vi "曲线对齐.vi"() -> ()   [LabVIEW 2015]
uses:
  <vilib>/Utility/miscctls.llb/LVCursorListTypeDef.ctl
  <vilib>/Utility/file.llb/Read Delimited Spreadsheet (DBL).vi
  <vilib>/gmath/NI_Gmath.lvlib
panel:
  in  "重采样间隔":dbl=0.1 format="%.3fs"
  in  "取消修改":bool
  in  "当前编辑曲线":T1
  in  "确认修改":bool
  in  "功能选择":T2
  in  "加载数据":bool
  out "曲线对齐":cluster{"理论时间":dbl[], "力":dbl[]}[](graph)
  out "all rows 2":dbl[][](array[numeric]) caption="所有行"
  in  "理论曲线路径":path=path "D:/曲线处理/理论1.csv" caption="理论"
  out "all rows":dbl[][](array[numeric]) caption="所有行"
  in  "测量曲线路径":path=path "D:/曲线处理/实测1.csv" caption="实际"
  in  "Enqueue Element":bool caption="元素入队列"
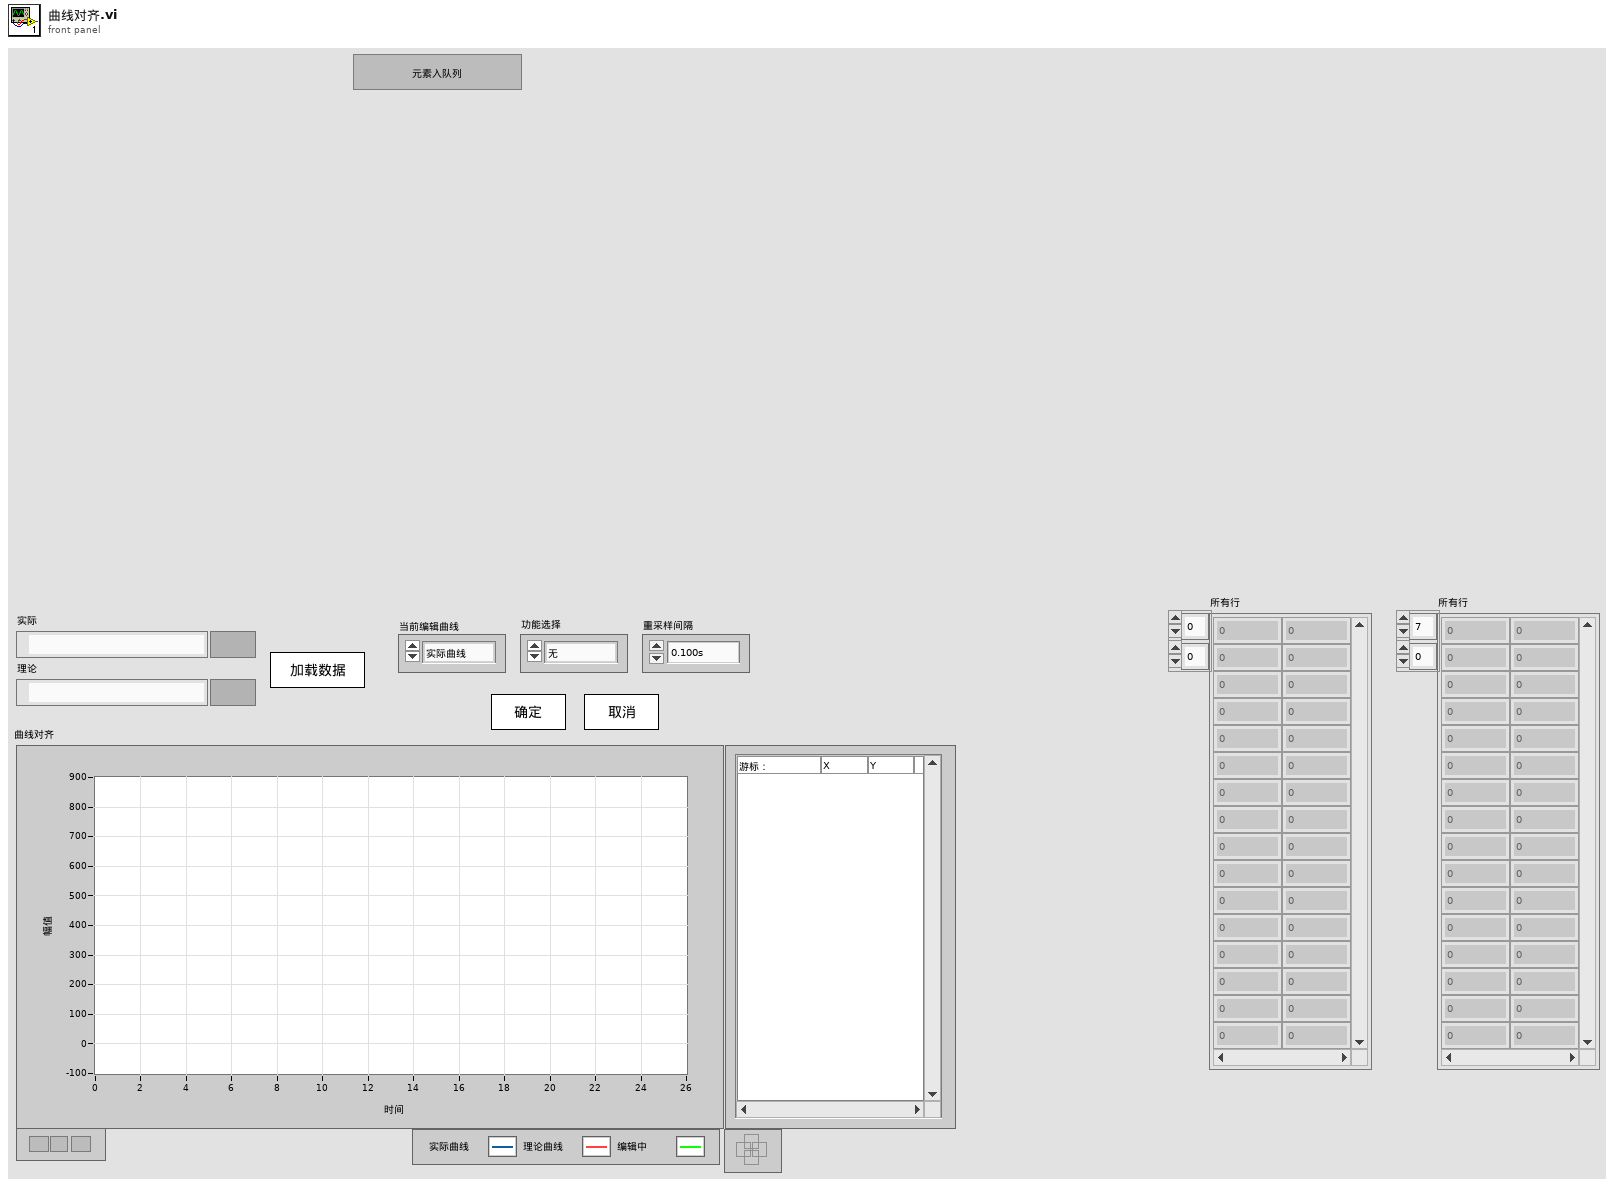
[diagram p1: front panel]
types:
  T1 = typedef "曲线选择.ctl" = enum16{"实际曲线", "理论曲线", "编辑中曲线", "实际曲线原始值", "理论曲线原始值"}
  T2 = typedef "功能选择.ctl" = enum16{"无", "缩放曲线", "剪裁曲线", "对齐曲线", "初始值置0", "重采样", "曲线平滑"}
  T3 = typedef "LVCursorListTypeDef.ctl" = cluster{"Name":string, "Color":u32, "Style":u8, "Point Style":u8, "Name Visible":bool, "Allow Drag":bool, "Cursor Mode":u32, "Plot":i32, "Index":i32, "Position":cluster{"X":dbl, "Y":dbl}, "X Scale":u32, "Y Scale":u32, "Watch Plots":i32[], "Watch All Plots":bool, "Plot Area":i32, "Label Offset":cluster{"X":dbl, "Y":dbl}}[]
  T4 = cluster{"Name":string, "Color":u32, "Style":u8, "Point Style":u8, "Name Visible":bool, "Allow Drag":bool, "Cursor Mode":u32, "Plot":i32, "Index":i32, "Position":cluster{"X":dbl, "Y":dbl}, "X Scale":u32, "Y Scale":u32, "Watch Plots":i32[], "Watch All Plots":bool, "Plot Area":i32, "Label Offset":cluster{"X":dbl, "Y":dbl}}
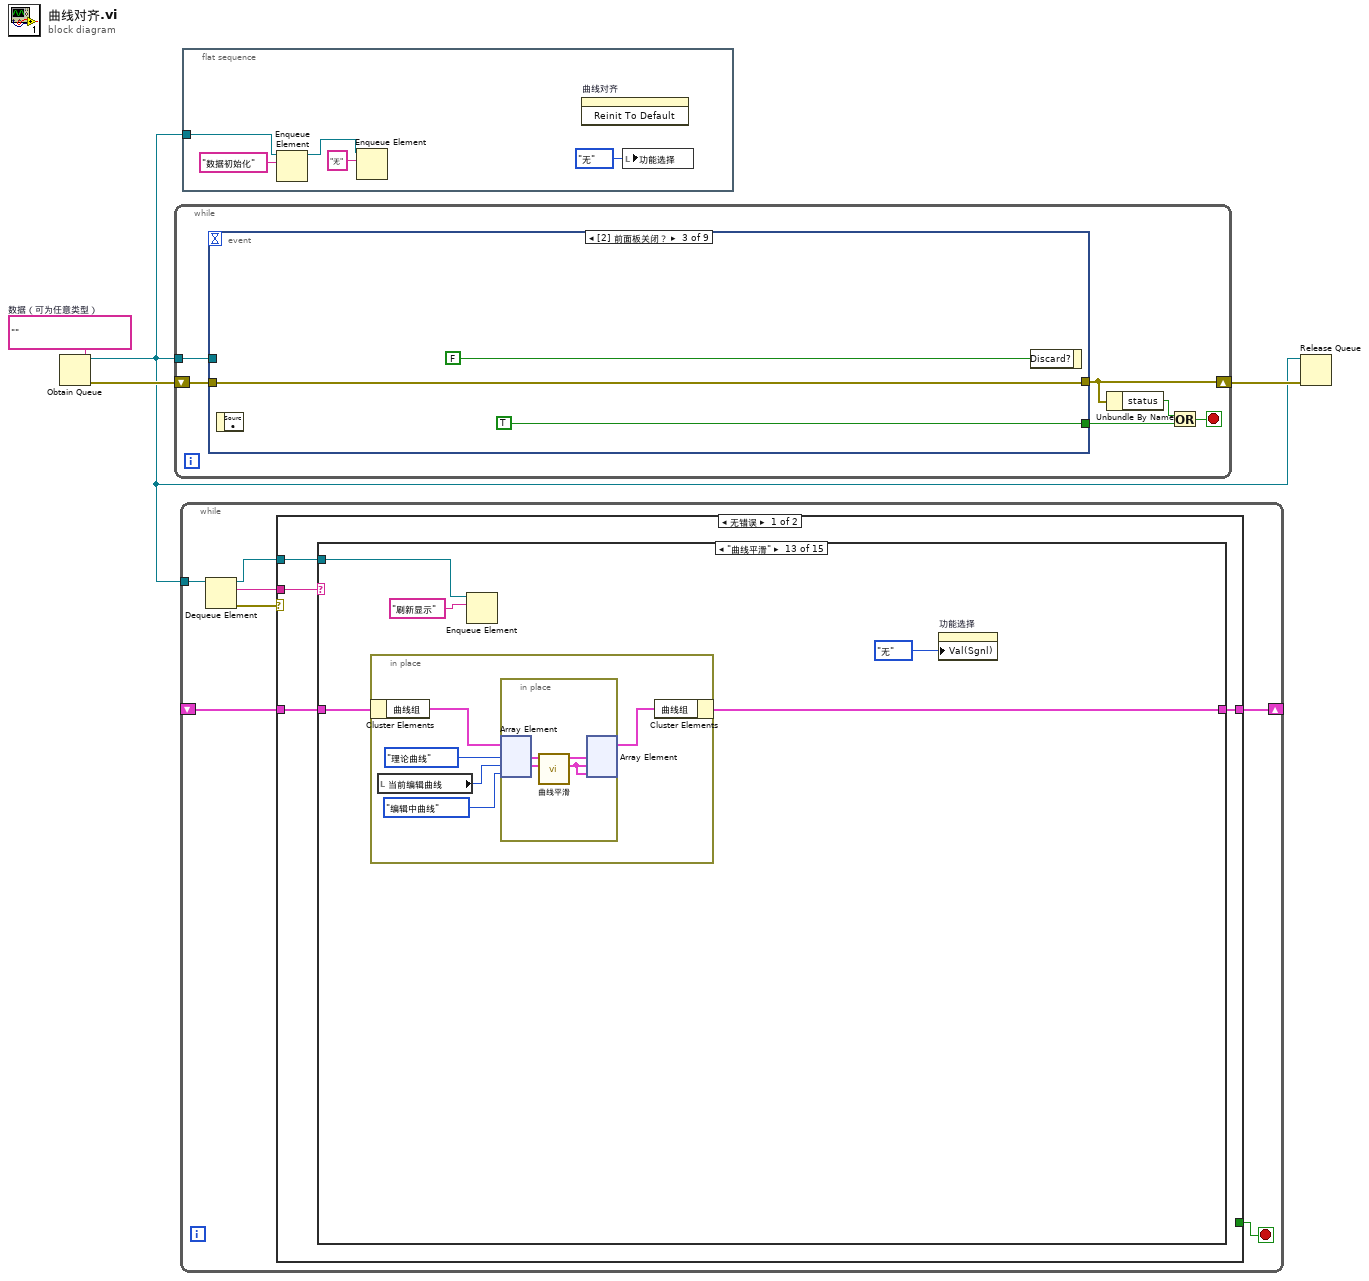
[diagram p0: block diagram]
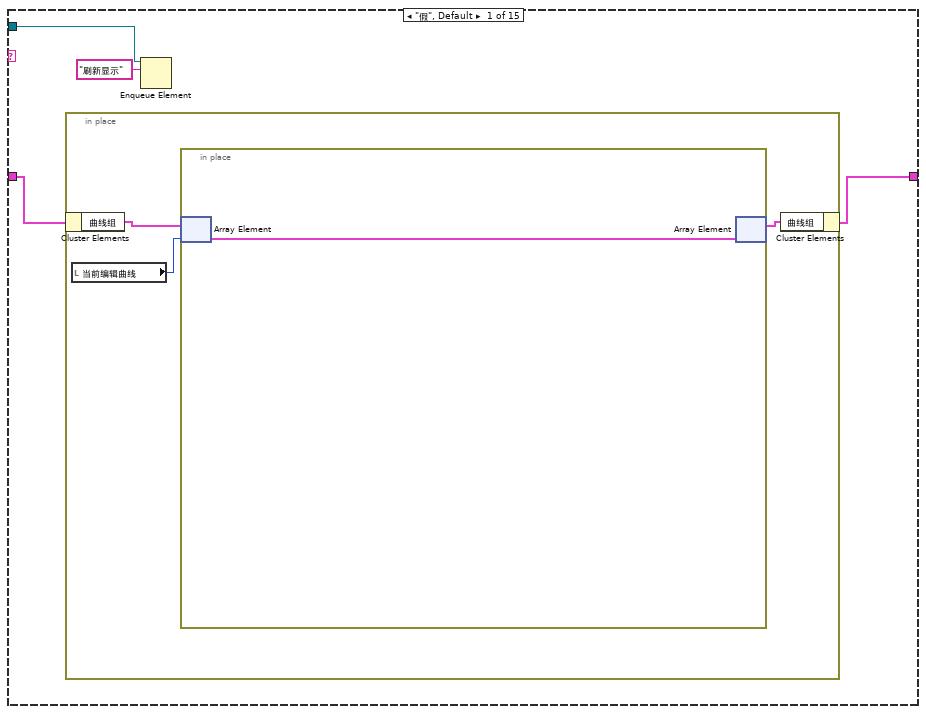
[diagram p2: hidden frame]
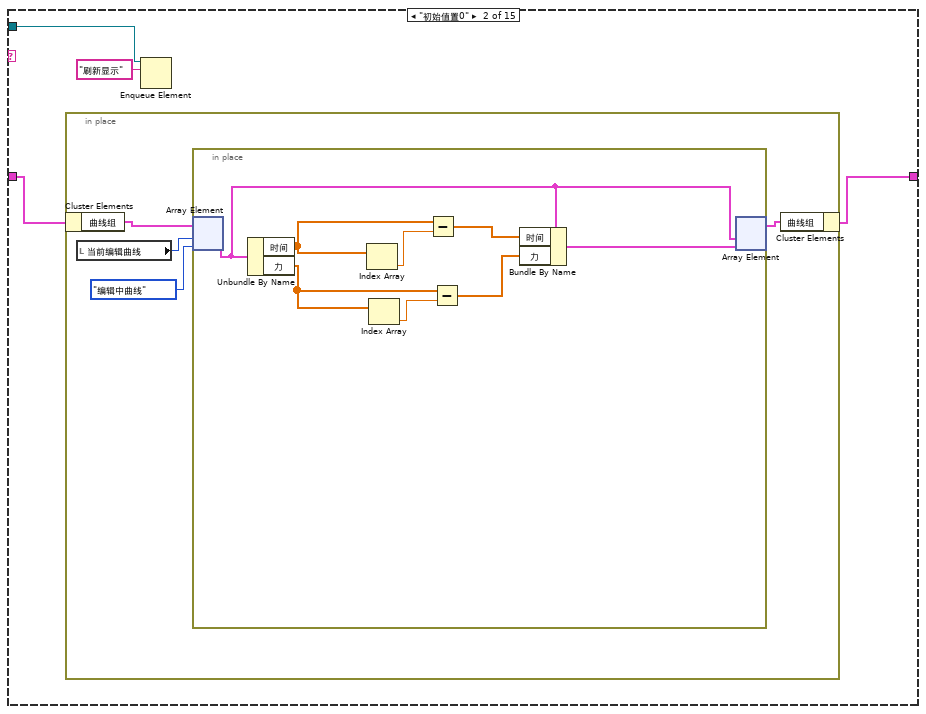
[diagram p3: hidden frame]
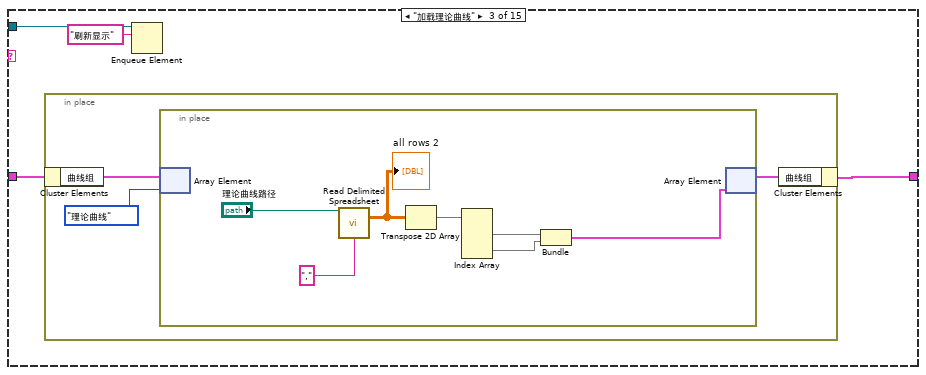
[diagram p4: hidden frame]
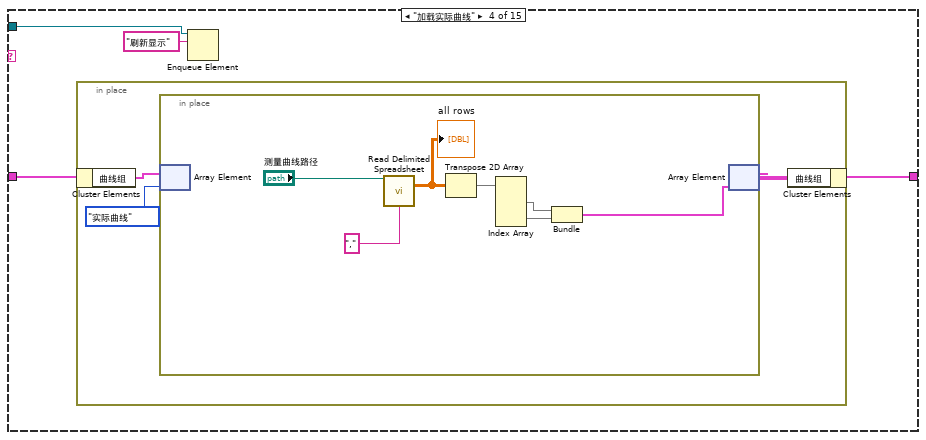
[diagram p5: hidden frame]
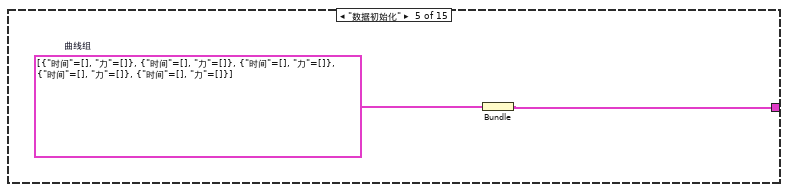
[diagram p6: hidden frame]
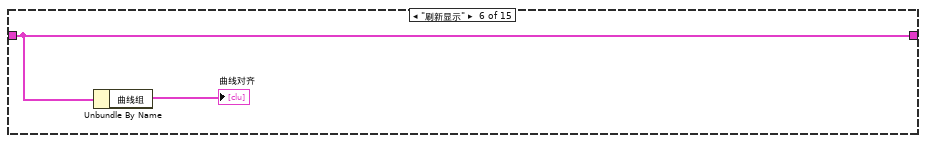
[diagram p7: hidden frame]
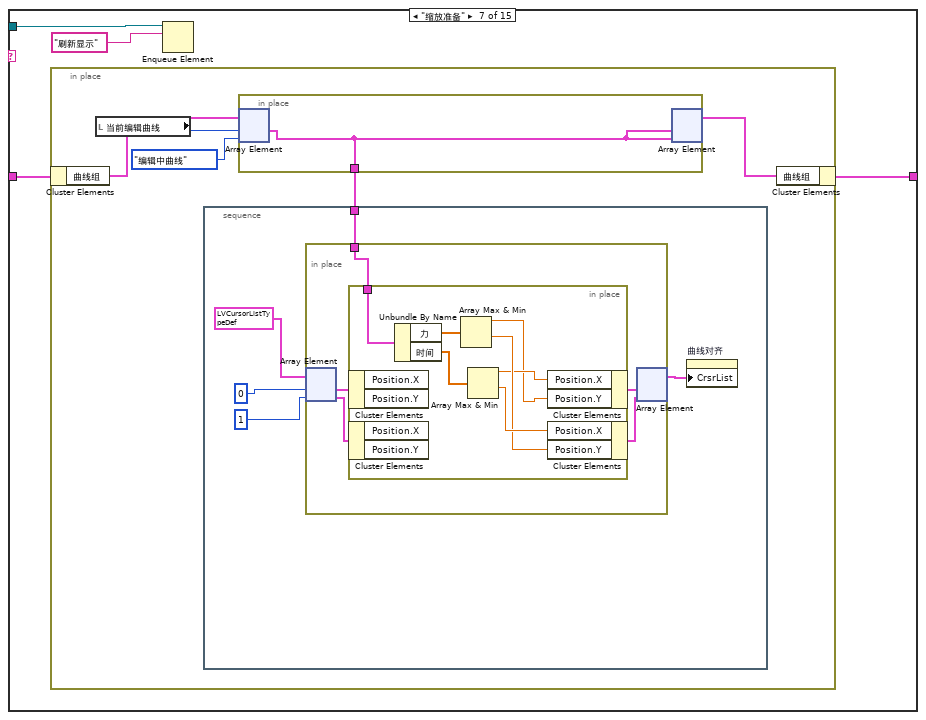
[diagram p8: hidden frame]
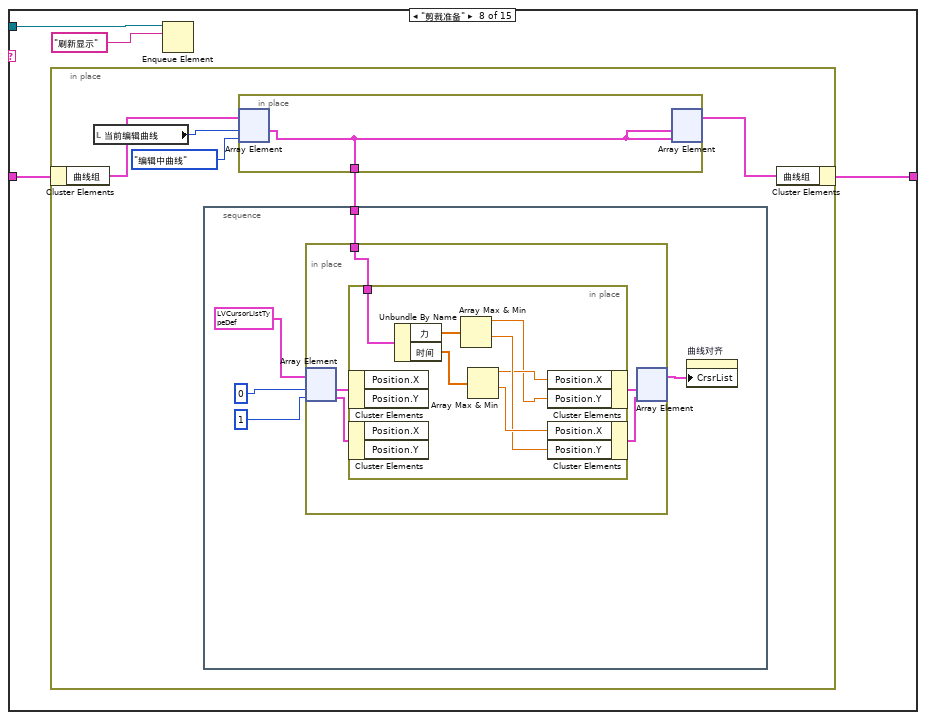
[diagram p9: hidden frame]
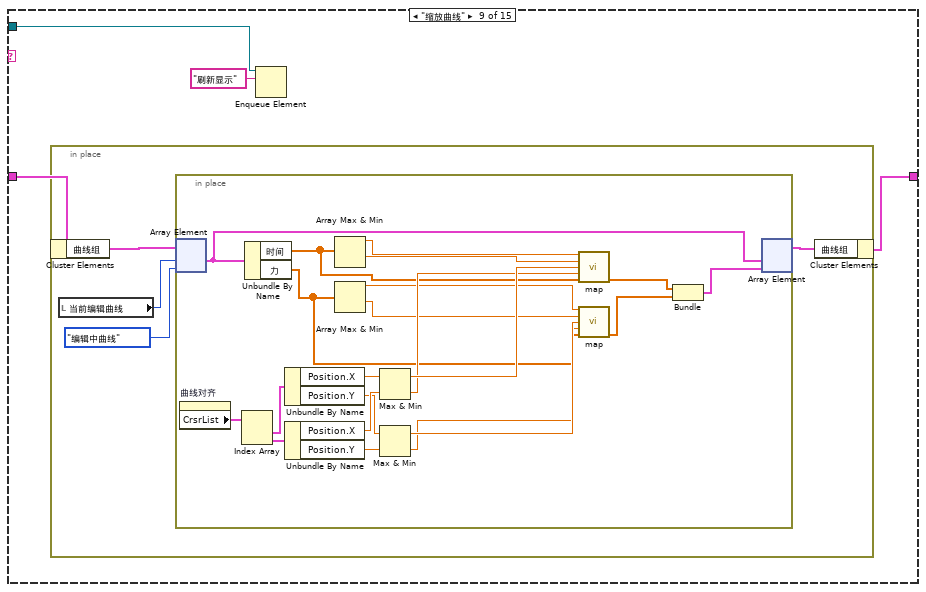
[diagram p10: hidden frame]
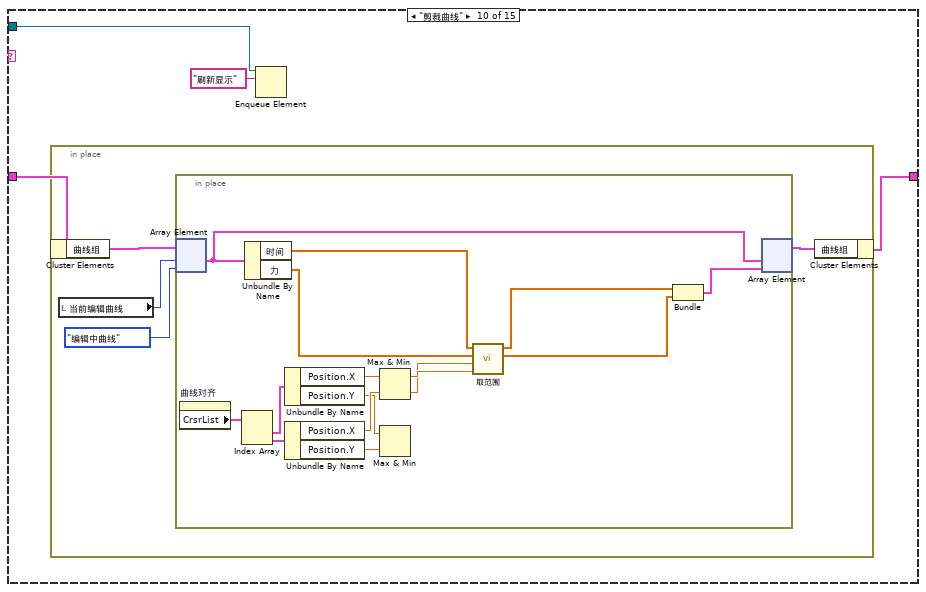
[diagram p11: hidden frame]
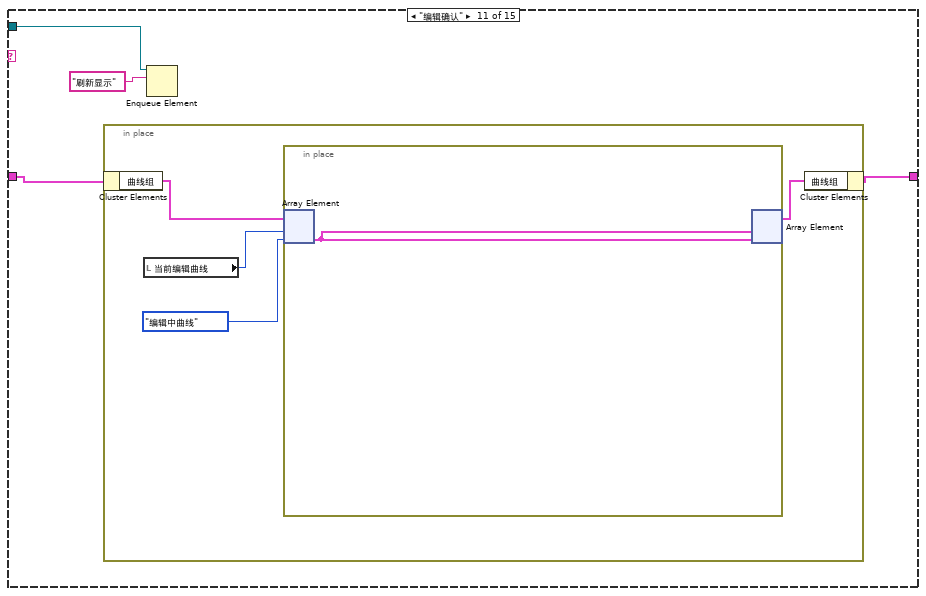
[diagram p12: hidden frame]
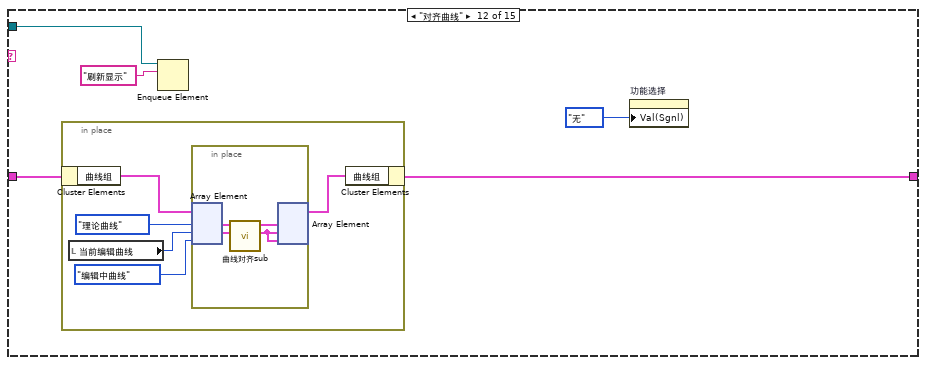
[diagram p13: hidden frame]
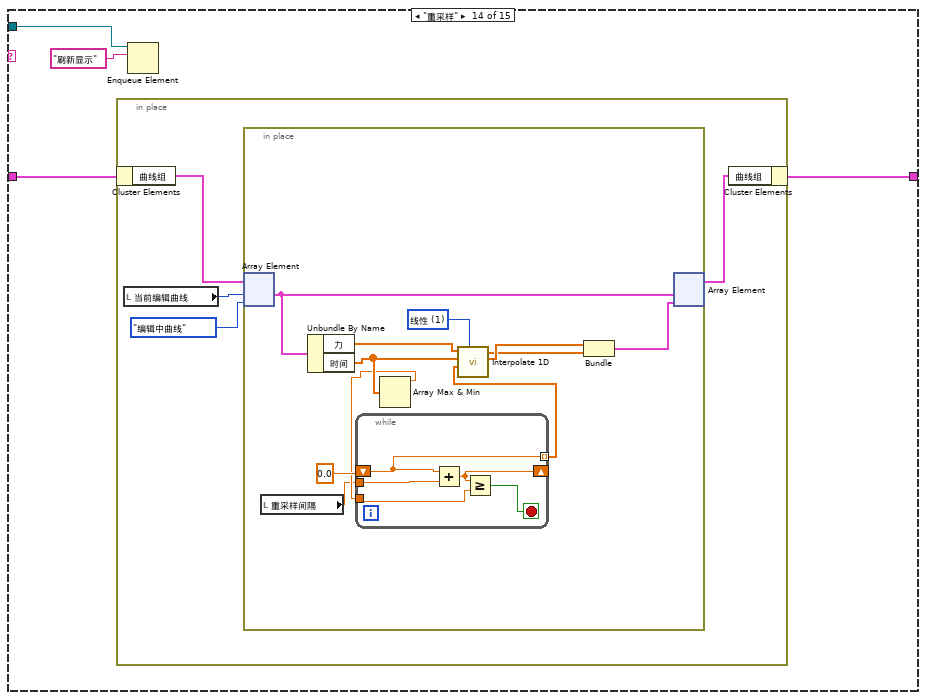
[diagram p14: hidden frame]
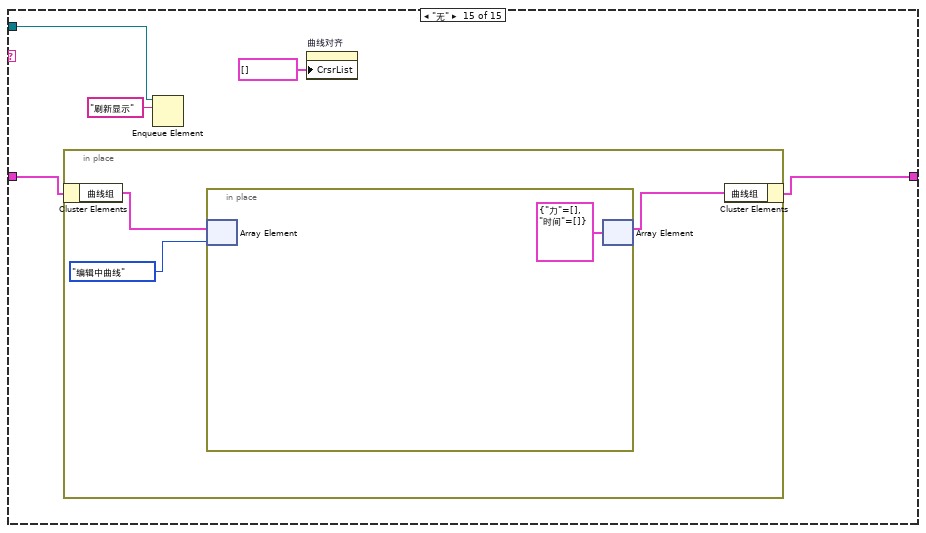
[diagram p15: hidden frame]
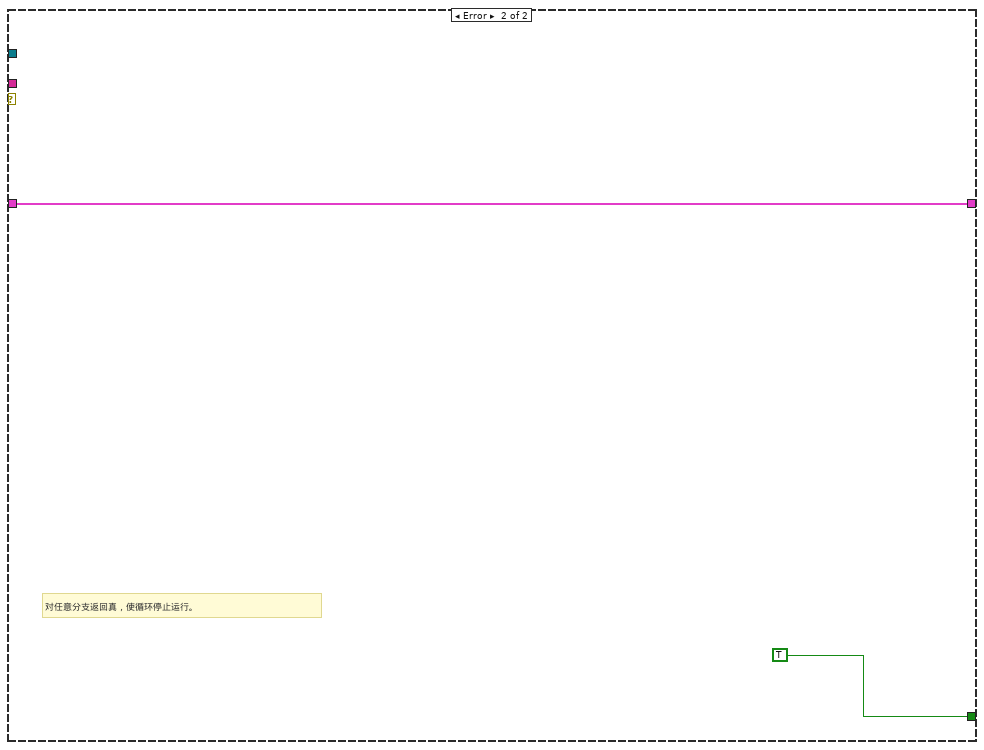
[diagram p16: hidden frame]
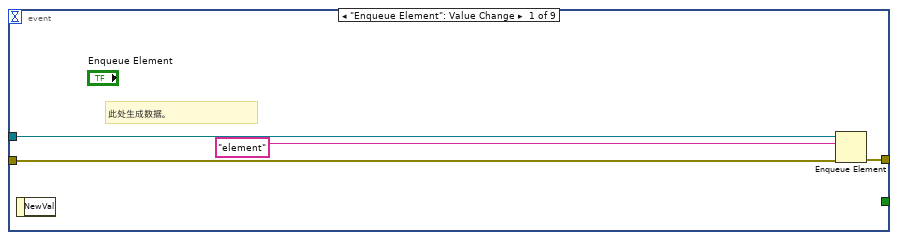
[diagram p17: hidden frame]
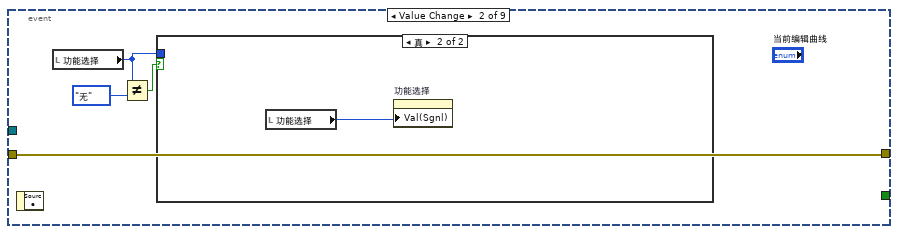
[diagram p18: hidden frame]
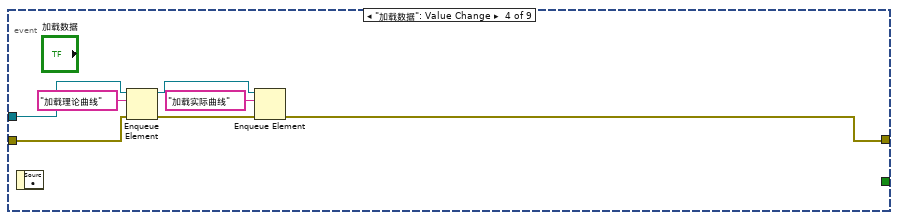
[diagram p20: hidden frame]
diagram:
  w4 = ""  # 数据（可为任意类型）
  n1 = Obtain Queue(element data type=w4) -> (queue out=w1:refnum<queue>, error out=w2:errorcluster)  [unwired: 4 in, 1 out]
  n2 = while {
    shift-right: [w6] -> w3
    shift-left: w2 -> [w9]
    tunnel: w1 -> [w10]
    stop <- w7 stop-if-true
    n3 = event shown="[2] 前面板关闭？" {
      selector: _ -> [_ _ _ _ _ _ _ _ _]
      dyn-events: _ -> [_ _ _ _ _ _ _ _ _]
      timeout: _ -> [_ _ _ _ _ _ _ _ _]
      tunnel: w10 -> [w14 _ _ w27 w33 _ w43 w47 w64]
      tunnel: w9 -> [w13 w18 w22 w24 w34 w38 w44 w49 w66]
      tunnel: [w12 w18 w22 w23 w34 w37 w44 w49 w66] -> w6
      tunnel: [_ _ TRUE ("stop") _ _ _ _ _ _] -> w8
      event "Enqueue Element": Value Change {
        # "此处生成数据。"
        n4 = event-data() -> ()  [unwired: 1 in, 1 out]
        n5 = Enqueue Element(queue=w14, element="element", error in (no error)=w13) -> (error out=w12:errorcluster)  [unwired: 1 in, 2 out]
      }
      event Value Change {
        n6 = event-data() -> ()  [unwired: 1 in, 1 out]
        n7 = local read "功能选择"() -> (w15:T2)
        n8 = Not Equal?(x=w15, y=功能选择."无") -> (x != y?=w17:bool)
        n9 = case shown="真" w17 {
          tunnel: w15 -> [_ _]
          frame False {
          }
          frame True {
            n10 = local read "功能选择"() -> (w19:T2)
            n11 = property on="功能选择" class="Enum (严格)"("Val(Sgnl)"=w19) -> ()  [unwired: 2 in, 2 out]
          }
        }
      }
      event Panel Close? {
        n12 = event-data() -> ()  [unwired: 1 in, 1 out]
        n13 = event-data("Discard?"=FALSE ("放弃？")) -> ()  [unwired: 1 in, 1 out]
      }
      event "加载数据": Value Change {
        n14 = event-data() -> ()  [unwired: 1 in, 1 out]
        n15 = Enqueue Element(queue=w27, element="加载理论曲线" ("元素"), error in (no error)=w24) -> (queue out=w26:refnum<queue>, error out=w25:errorcluster)  [unwired: 1 in, 1 out]
        n16 = Enqueue Element(queue=w26, element="加载实际曲线" ("元素"), error in (no error)=w25) -> (error out=w23:errorcluster)  [unwired: 1 in, 2 out]
      }
      event "确认修改": Value Change {
        n17 = event-data() -> ()  [unwired: 1 in, 1 out]
        n18 = local read "功能选择"() -> (w32:T2)
        n19 = Not Equal?(x=w32, y=功能选择."无") -> (x != y?=w31:bool)
        n20 = case shown="真" w31 {
          tunnel: w33 -> [_ w35]
          frame False {
          }
          frame True {
            n21 = Enqueue Element(queue=w35, element="编辑确认" ("元素")) -> ()  [unwired: 2 in, 3 out]
          }
        }
      }
      event "取消修改": Value Change {
        n22 = event-data() -> ()  [unwired: 1 in, 1 out]
        n23 = property on="功能选择" class="Enum (严格)"(error in=w38, "Val(Sgnl)"=功能选择."无" ("值(信号)")) -> (error out=w37:errorcluster)  [unwired: 1 in, 1 out]
      }
      event "重采样间隔": Value Change {
        n24 = event-data() -> ()  [unwired: 1 in, 1 out]
        n25 = local read "功能选择"() -> (w41:T2)
        n26 = Equal?(x=w41, y=功能选择."重采样") -> (x = y?=w42:bool)
        n27 = case shown="真" w42 {
          tunnel: w43 -> [_ w45]
          frame False {
          }
          frame True {
            n28 = Enqueue Element(queue=w45, element="重采样" ("元素")) -> ()  [unwired: 2 in, 3 out]
          }
        }
      }
      event Value Change {
        n29 = event-data() -> ("NewVal"=w48:T2)  [unwired: 1 in]
        n30 = case shown="\"曲线平滑\"" w48 {
          tunnel: w47 -> [w50 w53 w54 w56 w58 w61 w62]
          frame "缩放曲线", Default {
            n31 = Enqueue Element(queue=w50, element="缩放准备" ("元素")) -> ()  [unwired: 2 in, 3 out]
          }
          frame "无" {
            n32 = Enqueue Element(queue=w53, element="无" ("元素")) -> ()  [unwired: 2 in, 3 out]
          }
          frame "剪裁曲线" {
            n33 = Enqueue Element(queue=w54, element="剪裁准备" ("元素")) -> ()  [unwired: 2 in, 3 out]
          }
          frame "对齐曲线" {
            n34 = Enqueue Element(queue=w56, element="对齐曲线" ("元素")) -> ()  [unwired: 2 in, 3 out]
          }
          frame "初始值置0" {
            n35 = Enqueue Element(queue=w58, element="初始值置0" ("元素")) -> ()  [unwired: 2 in, 3 out]
          }
          frame "重采样" {
            n36 = Enqueue Element(queue=w61, element="重采样" ("元素")) -> ()  [unwired: 2 in, 3 out]
          }
          frame "曲线平滑" {
            n37 = Enqueue Element(queue=w62, element="曲线平滑" ("元素")) -> ()  [unwired: 2 in, 3 out]
          }
        }
      }
      event "曲线对齐": Cursor Move {
        n38 = event-data() -> ()  [unwired: 1 in, 8 out]
        n39 = local read "功能选择"() -> (w65:T2)
        n40 = case shown="\"无\", 默认" w65 {
          tunnel: w64 -> [_ w67 w69]
          frame "无", Default {
          }
          frame "缩放曲线" {
            n41 = Enqueue Element(queue=w67, element="缩放曲线" ("元素")) -> ()  [unwired: 2 in, 3 out]
          }
          frame "剪裁曲线" {
            n42 = Enqueue Element(queue=w69, element="剪裁曲线" ("元素")) -> ()  [unwired: 2 in, 3 out]
          }
        }
      }
    }
    n43 = Unbundle By Name(w6) -> ("status"=w5:bool)
    n44 = Or(x=w5, y=w8) -> (x .or. y?=w7:bool)
  }
  n45 = while {
    tunnel: w1 -> [w72]
    shift-right: [w74] -> _
    shift-left: _ -> [w73]
    stop <- w75 stop-if-true
    n46 = Dequeue Element(queue=w72) -> (queue out=w71:refnum<queue>, element=w76:string, error out=w77:errorcluster)  [unwired: 2 in, 1 out]
    n47 = case shown="无错误" w77 {
      tunnel: w76 -> [w81 _]
      tunnel: [_ TRUE] -> w75
      tunnel: [w78 w314] -> w74
      tunnel: w73 -> [w80 w314]
      tunnel: w71 -> [w79 _]
      frame No Error {
        n48 = case shown="\"曲线平滑\"" w81 {
          tunnel: [w82 w90 w109 w123 w135 w137 w138 w165 w192 w221 w244 w256 w270 w283 w305] -> w78
          tunnel: w80 -> [w83 w91 w106 w120 _ w137 w139 w166 w193 w222 w245 w257 w271 w284 w306]
          tunnel: w79 -> [w84 w92 w108 w121 _ _ w140 w167 w194 w223 w246 w254 w268 w281 w307]
          frame "假", Default {
            n49 = in-place {
              n50 = in-place-cluster #1(w83) -> ("曲线组"=w88:cluster{"时间":dbl[], "力":dbl[]}[])
              n51 = local read "当前编辑曲线"() -> (w86:T1)
              n52 = in-place {
                n53 = in-place-array #2(w88, w86) -> (w89:cluster{"时间":dbl[], "力":dbl[]})
                n54 = in-place-array #2(w89) -> (w87:cluster{"时间":dbl[], "力":dbl[]}[])  [unwired: 1 out]
              }
              n55 = in-place-cluster #1("曲线组"=w87) -> (w82:cluster{"曲线组":cluster{"时间":dbl[], "力":dbl[]}[]})
            }
            n56 = Enqueue Element(queue=w84, element="刷新显示" ("元素")) -> ()  [unwired: 2 in, 3 out]
          }
          frame "初始值置0" {
            n57 = in-place {
              n58 = in-place-cluster #3(w91) -> ("曲线组"=w97:cluster{"时间":dbl[], "力":dbl[]}[])
              n59 = local read "当前编辑曲线"() -> (w95:T1)
              n60 = in-place {
                n61 = in-place-array #4(w97, w95, 曲线选择."编辑中曲线" ("当前编辑曲线")) -> (w99:cluster{"时间":dbl[], "力":dbl[]})  [unwired: 1 out]
                n62 = Unbundle By Name(w99) -> ("时间"=w105:dbl[], "力"=w103:dbl[])
                n63 = Index Array(array=w105) -> (element=w104:dbl)  [unwired: 1 in]
                n64 = Index Array(array=w103) -> (element=w102:dbl)  [unwired: 1 in]
                n65 = Subtract(x=w105, y=w104) -> (x-y=w101:dbl[])
                n66 = Subtract(x=w103, y=w102) -> (x-y=w100:dbl[])
                n67 = Bundle By Name(cluster=w99, "时间"=w101, "力"=w100) -> (w98:cluster{"时间":dbl[], "力":dbl[]})
                n68 = in-place-array #4(w99, w98) -> (w96:cluster{"时间":dbl[], "力":dbl[]}[])  [unwired: 2 out]
              }
              n69 = in-place-cluster #3("曲线组"=w96) -> (w90:cluster{"曲线组":cluster{"时间":dbl[], "力":dbl[]}[]})
            }
            n70 = Enqueue Element(queue=w92, element="刷新显示" ("元素")) -> ()  [unwired: 2 in, 3 out]
          }
          frame "加载理论曲线" {
            n71 = in-place {
              n72 = in-place-cluster #5(w106) -> ("曲线组"=w112:cluster{"时间":dbl[], "力":dbl[]}[])
              n73 = in-place {
                n74 = in-place-array #6(w112, 曲线选择."理论曲线" ("当前编辑曲线")) -> ()  [unwired: 1 out]
                n75 = call-poly <vilib>:"Read Delimited Spreadsheet.vi"("file path (dialog if empty)"="理论曲线路径", "delimiter (\\t)"="," ("delimiter (\\t)")) -> ("all rows"=w116:dbl[][])  [unwired: 8 in, 5 out]
                "all rows 2" <- w116
                n76 = Transpose 2D Array(2D array=w116) -> (transposed array=w117:dbl[][])
                n77 = Index Array(array=w117) -> (element #1=w115:dbl[], element #2=w114:dbl[])  [unwired: 4 in]
                n78 = Bundle(w115, w114) -> (w113:cluster{dbl[], dbl[]})  [unwired: 1 in]
                n79 = in-place-array #6(w113) -> (w111:cluster{"时间":dbl[], "力":dbl[]}[])  [unwired: 1 out]
              }
              n80 = in-place-cluster #5("曲线组"=w111) -> (w109:cluster{"曲线组":cluster{"时间":dbl[], "力":dbl[]}[]})
            }
            n81 = Enqueue Element(queue=w108, element="刷新显示" ("元素")) -> ()  [unwired: 2 in, 3 out]
          }
          frame "加载实际曲线" {
            n82 = in-place {
              n83 = in-place-cluster #7(w120) -> ("曲线组"=w126:cluster{"时间":dbl[], "力":dbl[]}[])
              n84 = in-place {
                n85 = in-place-array #8(w126, 曲线选择."实际曲线") -> ()  [unwired: 1 out]
                n86 = call-poly <vilib>:"Read Delimited Spreadsheet.vi"("file path (dialog if empty)"="测量曲线路径", "delimiter (\\t)"="," ("delimiter (\\t)")) -> ("all rows"=w132:dbl[][])  [unwired: 8 in, 5 out]
                "all rows" <- w132
                n87 = Transpose 2D Array(2D array=w132) -> (transposed array=w133:dbl[][])
                n88 = Index Array(array=w133) -> (element #1=w129:dbl[], element #2=w128:dbl[])  [unwired: 4 in]
                n89 = Bundle(w129, w128) -> (w127:cluster{dbl[], dbl[]})  [unwired: 1 in]
                n90 = in-place-array #8(w127) -> (w124:cluster{"时间":dbl[], "力":dbl[]}[])  [unwired: 1 out]
              }
              n91 = in-place-cluster #7("曲线组"=w124) -> (w123:cluster{"曲线组":cluster{"时间":dbl[], "力":dbl[]}[]})
            }
            n92 = Enqueue Element(queue=w121, element="刷新显示" ("元素")) -> ()  [unwired: 2 in, 3 out]
          }
          frame "数据初始化" {
            w134 = cluster{"时间":dbl[], "力":dbl[]}[] [{"时间"=[], "力"=[]}, {"时间"=[], "力"=[]}, {"时间"=[], "力"=[]}, {"时间"=[], "力"=[]}, {"时间"=[], "力"=[]}]  # 曲线组
            n93 = Bundle("曲线组"=w134) -> (w135:cluster{"曲线组":cluster{"时间":dbl[], "力":dbl[]}[]})  [unwired: 1 in]
          }
          frame "刷新显示" {
            n94 = Unbundle By Name(w137) -> ("曲线组"=→"曲线对齐":cluster{"时间":dbl[], "力":dbl[]}[])
          }
          frame "缩放准备" {
            n95 = in-place {
              n96 = in-place-cluster #9(w139) -> ("曲线组"=w146:cluster{"时间":dbl[], "力":dbl[]}[])
              n97 = local read "当前编辑曲线"() -> (w142:T1)
              n98 = in-place {
                in-place-border: [w147] -> w143
                n99 = in-place-array #10(w146, w142, 曲线选择."编辑中曲线" ("当前编辑曲线")) -> (w147:cluster{"时间":dbl[], "力":dbl[]})  [unwired: 1 out]
                n100 = in-place-array #10(w147, w147) -> (w144:cluster{"时间":dbl[], "力":dbl[]}[])  [unwired: 2 out]
              }
              n101 = stacked-sequence {
                tunnel: w143 -> [w148]
                frame #0 {
                  n102 = in-place {
                    in-place-border: w148 -> [w153]
                    n103 = in-place-array #11(T3 [{"Name"="游标0", "Color"=16711680, "Style"=8, "Point Style"=13, "Name Visible"=FALSE, "Allow Drag"=TRUE, "Cursor Mode"=0, "Plot"=0, "Index"=0, "Position"={"X"=24.900169204737733, "Y"=876.3513513513514}, "X Scale"=0, "Y Scale"=0, "Watch Plots"=[], "Watch All Plots"=FALSE, "Plot Area"=0, "Label Offset"={"X"=0.0, "Y"=67.56756756756761}}, {"Name"="游标1", "Color"=16860, "Style"=8, "Point Style"=13, "Name Visible"=FALSE, "Allow Drag"=TRUE, "Cursor Mode"=0, "Plot"=0, "Index"=0, "Position"={"X"=-2.199661590524536, "Y"=1.3513513513513553}, "X Scale"=0, "Y Scale"=0, "Watch Plots"=[], "Watch All Plots"=FALSE, "Plot Area"=0, "Label Offset"={"X"=8.881784197001252e-16, "Y"=67.56756756756756}}] ("游标列表"), 0, 1) -> (w157:T4, w156:T4)
                    n104 = in-place {
                      in-place-border: w153 -> [w160]
                      n105 = in-place-cluster #12(w157) -> ()  [unwired: 2 out]
                      n106 = in-place-cluster #13(w156) -> ()  [unwired: 2 out]
                      n107 = Unbundle By Name(w160) -> ("力"=w159:dbl[], "时间"=w158:dbl[])
                      n108 = Array Max & Min(array=w159) -> (max value=w161:dbl, min value=w163:dbl)  [unwired: 2 out]
                      n109 = Array Max & Min(array=w158) -> (max value=w162:dbl, min value=w164:dbl)  [unwired: 2 out]
                      n110 = in-place-cluster #12("Position.X"=w162, "Position.Y"=w161) -> (w155:T4)
                      n111 = in-place-cluster #13("Position.X"=w164, "Position.Y"=w163) -> (w154:T4)
                    }
                    n112 = in-place-array #11(w155, w154) -> (w149:T3)  [unwired: 2 out]
                  }
                  n113 = property on="曲线对齐" class="XYGraph (严格)"("CrsrList"=w149) -> ()  [unwired: 2 in, 2 out]
                }
              }
              n114 = in-place-cluster #9("曲线组"=w144) -> (w138:cluster{"曲线组":cluster{"时间":dbl[], "力":dbl[]}[]})
            }
            n115 = Enqueue Element(queue=w140, element="刷新显示" ("元素")) -> ()  [unwired: 2 in, 3 out]
          }
          frame "剪裁准备" {
            n116 = in-place {
              n117 = in-place-cluster #14(w166) -> ("曲线组"=w173:cluster{"时间":dbl[], "力":dbl[]}[])
              n118 = local read "当前编辑曲线"() -> (w169:T1)
              n119 = in-place {
                in-place-border: [w174] -> w170
                n120 = in-place-array #15(w173, w169, 曲线选择."编辑中曲线" ("当前编辑曲线")) -> (w174:cluster{"时间":dbl[], "力":dbl[]})  [unwired: 1 out]
                n121 = in-place-array #15(w174, w174) -> (w171:cluster{"时间":dbl[], "力":dbl[]}[])  [unwired: 2 out]
              }
              n122 = stacked-sequence {
                tunnel: w170 -> [w175]
                frame #0 {
                  n123 = in-place {
                    in-place-border: w175 -> [w180]
                    n124 = in-place-array #16(T3 [{"Name"="游标0", "Color"=16711680, "Style"=8, "Point Style"=13, "Name Visible"=FALSE, "Allow Drag"=TRUE, "Cursor Mode"=0, "Plot"=0, "Index"=0, "Position"={"X"=24.900169204737733, "Y"=876.3513513513514}, "X Scale"=0, "Y Scale"=0, "Watch Plots"=[], "Watch All Plots"=FALSE, "Plot Area"=0, "Label Offset"={"X"=0.0, "Y"=67.56756756756761}}, {"Name"="游标1", "Color"=16860, "Style"=8, "Point Style"=13, "Name Visible"=FALSE, "Allow Drag"=TRUE, "Cursor Mode"=0, "Plot"=0, "Index"=0, "Position"={"X"=-2.199661590524536, "Y"=1.3513513513513553}, "X Scale"=0, "Y Scale"=0, "Watch Plots"=[], "Watch All Plots"=FALSE, "Plot Area"=0, "Label Offset"={"X"=8.881784197001252e-16, "Y"=67.56756756756756}}] ("游标列表"), 0, 1) -> (w184:T4, w183:T4)
                    n125 = in-place {
                      in-place-border: w180 -> [w187]
                      n126 = in-place-cluster #17(w184) -> ()  [unwired: 2 out]
                      n127 = in-place-cluster #18(w183) -> ()  [unwired: 2 out]
                      n128 = Unbundle By Name(w187) -> ("力"=w186:dbl[], "时间"=w185:dbl[])
                      n129 = Array Max & Min(array=w186) -> (max value=w188:dbl, min value=w190:dbl)  [unwired: 2 out]
                      n130 = Array Max & Min(array=w185) -> (max value=w189:dbl, min value=w191:dbl)  [unwired: 2 out]
                      n131 = in-place-cluster #17("Position.X"=w189, "Position.Y"=w188) -> (w182:T4)
                      n132 = in-place-cluster #18("Position.X"=w191, "Position.Y"=w190) -> (w181:T4)
                    }
                    n133 = in-place-array #16(w182, w181) -> (w176:T3)  [unwired: 2 out]
                  }
                  n134 = property on="曲线对齐" class="XYGraph (严格)"("CrsrList"=w176) -> ()  [unwired: 2 in, 2 out]
                }
              }
              n135 = in-place-cluster #14("曲线组"=w171) -> (w165:cluster{"曲线组":cluster{"时间":dbl[], "力":dbl[]}[]})
            }
            n136 = Enqueue Element(queue=w167, element="刷新显示" ("元素")) -> ()  [unwired: 2 in, 3 out]
          }
          frame "缩放曲线" {
            n137 = in-place {
              n138 = in-place-cluster #19(w193) -> ("曲线组"=w199:cluster{"时间":dbl[], "力":dbl[]}[])
              n139 = local read "当前编辑曲线"() -> (w198:T1)
              n140 = in-place {
                n141 = in-place-array #20(w199, w198, 曲线选择."编辑中曲线" ("当前编辑曲线")) -> (w202:cluster{"时间":dbl[], "力":dbl[]})  [unwired: 1 out]
                n142 = property on="曲线对齐" class="XYGraph (严格)"() -> ("CrsrList"=w220:T3)  [unwired: 2 in, 2 out]
                n143 = Index Array(array=w220) -> (element #1=w219:T4, element #2=w218:T4)  [unwired: 2 in]
                n144 = Unbundle By Name(w202) -> ("时间"=w201:dbl[], "力"=w200:dbl[])
                n145 = Unbundle By Name(w219) -> ("Position.X"=w217:dbl, "Position.Y"=w215:dbl)
                n146 = Unbundle By Name(w218) -> ("Position.X"=w216:dbl, "Position.Y"=w214:dbl)
                n147 = Array Max & Min(array=w201) -> (max value=w213:dbl, min value=w212:dbl)  [unwired: 2 out]
                n148 = Array Max & Min(array=w200) -> (max value=w209:dbl, min value=w208:dbl)  [unwired: 2 out]
                n149 = Max & Min(x=w217, y=w216) -> (max(x,y)=w211:dbl, min(x,y)=w210:dbl)
                n150 = Max & Min(x=w215, y=w214) -> (max(x,y)=w207:dbl, min(x,y)=w206:dbl)
                n151 = call "map.vi"("inmax"=w213, "inmin"=w212, "outmax"=w211, "outmin"=w210, "in"=w201) -> ("out"=w205:dbl[])  [unwired: 10 in]
                n152 = call "map.vi"("inmax"=w209, "inmin"=w208, "outmax"=w207, "outmin"=w206, "in"=w200) -> ("out"=w204:dbl[])  [unwired: 10 in]
                n153 = Bundle("out"=w205, "out"=w204) -> (w203:cluster{"out":dbl[], "out":dbl[]})  [unwired: 1 in]
                n154 = in-place-array #20(w202, w203) -> (w196:cluster{"时间":dbl[], "力":dbl[]}[])  [unwired: 2 out]
              }
              n155 = in-place-cluster #19("曲线组"=w196) -> (w192:cluster{"曲线组":cluster{"时间":dbl[], "力":dbl[]}[]})
            }
            n156 = Enqueue Element(queue=w194, element="刷新显示" ("元素")) -> ()  [unwired: 2 in, 3 out]
          }
          frame "剪裁曲线" {
            n157 = in-place {
              n158 = in-place-cluster #21(w222) -> ("曲线组"=w228:cluster{"时间":dbl[], "力":dbl[]}[])
              n159 = local read "当前编辑曲线"() -> (w227:T1)
              n160 = in-place {
                n161 = in-place-array #22(w228, w227, 曲线选择."编辑中曲线" ("当前编辑曲线")) -> (w236:cluster{"时间":dbl[], "力":dbl[]})  [unwired: 1 out]
                n162 = property on="曲线对齐" class="XYGraph (严格)"() -> ("CrsrList"=w243:T3)  [unwired: 2 in, 2 out]
                n163 = Index Array(array=w243) -> (element #1=w242:T4, element #2=w241:T4)  [unwired: 2 in]
                n164 = Unbundle By Name(w236) -> ("时间"=w233:dbl[], "力"=w232:dbl[])
                n165 = Unbundle By Name(w242) -> ("Position.X"=w240:dbl, "Position.Y"=w238:dbl)
                n166 = Unbundle By Name(w241) -> ("Position.X"=w239:dbl, "Position.Y"=w237:dbl)
                n167 = Max & Min(x=w240, y=w239) -> (max(x,y)=w235:dbl, min(x,y)=w234:dbl)
                n168 = Max & Min(x=w238, y=w237) -> ()  [unwired: 2 out]
                n169 = call "取范围.vi"("max"=w235, "min"=w234, "y"=w232, "x"=w233) -> ("y"=w230:dbl[], "x"=w231:dbl[])  [unwired: 6 in]
                n170 = Bundle("x"=w231, "y"=w230) -> (w229:cluster{"x":dbl[], "y":dbl[]})  [unwired: 1 in]
                n171 = in-place-array #22(w236, w229) -> (w225:cluster{"时间":dbl[], "力":dbl[]}[])  [unwired: 2 out]
              }
              n172 = in-place-cluster #21("曲线组"=w225) -> (w221:cluster{"曲线组":cluster{"时间":dbl[], "力":dbl[]}[]})
            }
            n173 = Enqueue Element(queue=w223, element="刷新显示" ("元素")) -> ()  [unwired: 2 in, 3 out]
          }
          frame "编辑确认" {
            n174 = in-place {
              n175 = in-place-cluster #23(w245) -> ("曲线组"=w251:cluster{"时间":dbl[], "力":dbl[]}[])
              n176 = local read "当前编辑曲线"() -> (w250:T1)
              n177 = in-place {
                n178 = in-place-array #24(w251, w250, 曲线选择."编辑中曲线" ("当前编辑曲线")) -> (w252:cluster{"时间":dbl[], "力":dbl[]})  [unwired: 1 out]
                n179 = in-place-array #24(w252, w252) -> (w248:cluster{"时间":dbl[], "力":dbl[]}[])  [unwired: 2 out]
              }
              n180 = in-place-cluster #23("曲线组"=w248) -> (w244:cluster{"曲线组":cluster{"时间":dbl[], "力":dbl[]}[]})
            }
            n181 = Enqueue Element(queue=w246, element="刷新显示" ("元素")) -> ()  [unwired: 2 in, 3 out]
          }
          frame "对齐曲线" {
            n182 = in-place {
              n183 = in-place-cluster #25(w257) -> ("曲线组"=w262:cluster{"时间":dbl[], "力":dbl[]}[])
              n184 = local read "当前编辑曲线"() -> (w259:T1)
              n185 = in-place {
                n186 = in-place-array #26(w262, 曲线选择."理论曲线" ("当前编辑曲线"), w259, 曲线选择."编辑中曲线" ("当前编辑曲线")) -> (w266:cluster{"时间":dbl[], "力":dbl[]}, w265:cluster{"时间":dbl[], "力":dbl[]})  [unwired: 1 out]
                n187 = call "曲线对齐sub.vi"("测量"=w265, "理论"=w266) -> ("实测"=w263:cluster{dbl[], dbl[]}, "理论"=w264:cluster{dbl[], dbl[]})  [unwired: 8 in]
                n188 = in-place-array #26(w264, w263, w263) -> (w260:cluster{"时间":dbl[], "力":dbl[]}[])  [unwired: 3 out]
              }
              n189 = in-place-cluster #25("曲线组"=w260) -> (w256:cluster{"曲线组":cluster{"时间":dbl[], "力":dbl[]}[]})
            }
            n190 = Enqueue Element(queue=w254, element="刷新显示" ("元素")) -> ()  [unwired: 2 in, 3 out]
            n191 = property on="功能选择" class="Enum (严格)"("Val(Sgnl)"=功能选择."无" ("功能选择")) -> ()  [unwired: 2 in, 2 out]
          }
          frame "曲线平滑" {
            n192 = in-place {
              n193 = in-place-cluster #27(w271) -> ("曲线组"=w276:cluster{"时间":dbl[], "力":dbl[]}[])
              n194 = local read "当前编辑曲线"() -> (w273:T1)
              n195 = in-place {
                n196 = in-place-array #28(w276, 曲线选择."理论曲线" ("当前编辑曲线"), w273, 曲线选择."编辑中曲线" ("当前编辑曲线")) -> (w280:cluster{"时间":dbl[], "力":dbl[]}, w279:cluster{"时间":dbl[], "力":dbl[]})  [unwired: 1 out]
                n197 = call "曲线平滑.vi"("测量"=w279, "理论"=w280) -> ("实测"=w277:cluster{dbl[], dbl[]}, "理论"=w278:cluster{dbl[], dbl[]})  [unwired: 8 in]
                n198 = in-place-array #28(w278, w277, w277) -> (w274:cluster{"时间":dbl[], "力":dbl[]}[])  [unwired: 3 out]
              }
              n199 = in-place-cluster #27("曲线组"=w274) -> (w270:cluster{"曲线组":cluster{"时间":dbl[], "力":dbl[]}[]})
            }
            n200 = Enqueue Element(queue=w268, element="刷新显示" ("元素")) -> ()  [unwired: 2 in, 3 out]
            n201 = property on="功能选择" class="Enum (严格)"("Val(Sgnl)"=功能选择."无" ("功能选择")) -> ()  [unwired: 2 in, 2 out]
          }
          frame "重采样" {
            n202 = in-place {
              n203 = in-place-cluster #29(w284) -> ("曲线组"=w288:cluster{"时间":dbl[], "力":dbl[]}[])
              n204 = local read "当前编辑曲线"() -> (w287:T1)
              n205 = in-place {
                w299 = 1 items=["最近", "线性", "样条", "cubic Hermite", "拉格朗日"] ("method")
                n206 = in-place-array #30(w288, w287, 曲线选择."编辑中曲线" ("当前编辑曲线")) -> (w290:cluster{"时间":dbl[], "力":dbl[]})  [unwired: 1 out]
                n207 = local read "重采样间隔"() -> (w289:dbl)
                n208 = Unbundle By Name(w290) -> ("力"=w298:dbl[], "时间"=w296:dbl[])
                n209 = Array Max & Min(array=w296) -> (max value=w295:dbl)  [unwired: 3 out]
                n210 = while {
                  shift-right: [w304] -> _
                  shift-left: 0.0 -> [w302]
                  tunnel: w295 -> [w303]
                  tunnel: [w302] -> w294 mode=indexing
                  tunnel: w289 -> [w300]
                  stop <- w301 stop-if-true
                  n211 = Add(x=w302, y=w300) -> (x+y=w304:dbl)
                  n212 = Greater Or Equal?(x=w304, y=w303) -> (x >= y?=w301:bool)
                }
                n213 = call <vilib>:"Interpolate 1D.vi"("method"=w299, "xi"=w294, "X"=w296, "Y"=w298) -> ("xi used"=w293:dbl[], "yi"=w292:dbl[])  [unwired: 5 in, 1 out]
                n214 = Bundle("xi used"=w293, "yi"=w292) -> (w291:cluster{"xi used":dbl[], "yi":dbl[]})  [unwired: 1 in]
                n215 = in-place-array #30(w290, w291) -> (w286:cluster{"时间":dbl[], "力":dbl[]}[])  [unwired: 2 out]
              }
              n216 = in-place-cluster #29("曲线组"=w286) -> (w283:cluster{"曲线组":cluster{"时间":dbl[], "力":dbl[]}[]})
            }
            n217 = Enqueue Element(queue=w281, element="刷新显示" ("元素")) -> ()  [unwired: 2 in, 3 out]
          }
          frame "无" {
            n218 = in-place {
              n219 = in-place-cluster #31(w306) -> ("曲线组"=w312:cluster{"时间":dbl[], "力":dbl[]}[])
              n220 = in-place {
                n221 = in-place-array #32(w312, 曲线选择."编辑中曲线" ("当前编辑曲线")) -> ()  [unwired: 1 out]
                n222 = in-place-array #32(cluster{"力":dbl[], "时间":dbl[]} {"力"=[], "时间"=[]} ("元素")) -> (w310:cluster{"时间":dbl[], "力":dbl[]}[])  [unwired: 1 out]
              }
              n223 = in-place-cluster #31("曲线组"=w310) -> (w305:cluster{"曲线组":cluster{"时间":dbl[], "力":dbl[]}[]})
            }
            n224 = Enqueue Element(queue=w307, element="刷新显示" ("元素")) -> ()  [unwired: 2 in, 3 out]
            n225 = property on="曲线对齐" class="XYGraph (严格)"("CrsrList"=T3 [] ("游标列表")) -> ()  [unwired: 2 in, 2 out]
          }
        }
      }
      frame Error {
        # "对任意分支返回真，使循环停止运行。"
      }
    }
  }
  n226 = flat-sequence {
    tunnel: w1 -> [w319]
    frame #0 {
      n227 = Enqueue Element(queue=w319, element="数据初始化" ("元素")) -> (queue out=w317:refnum<queue>)  [unwired: 2 in, 2 out]
      n228 = Enqueue Element(queue=w317, element="无" ("元素")) -> ()  [unwired: 2 in, 3 out]
      n229 = invoke on="曲线对齐" class="XYGraph (严格)" method="Reinit To Default"() -> ()  [unwired: 3 in, 3 out]
      n230 = local write "功能选择"(功能选择."无" ("功能选择")) -> ()
    }
  }
  n231 = Release Queue(queue=w1, error in (no error)=w3) -> ()  [unwired: 1 in, 3 out]
